vi "PixyCam_Open.vi"(4 "error in":errorcluster, 6 "SPI Bus":T4=enum."Invalid", 7 "Communication Mode":T5) -> (0 "error out":errorcluster, 3 "output cluster":T1)   [LabVIEW 2016, in "PixyCam_LabVIEW.lvlib"]
uses:
  PixyCam_LabVIEW.lvlib
  <vilib>/Rock Robotics/SystemInterfaces/spilib/spi_bus.ctl
  Private/PixyCam_CommMode.ctl
  Private/PixyCam_DevRef.ctl
  Private/PixyCam_SPI_DevRef.ctl
  <vilib>/Rock Robotics/WPI/SPI/WPI_SPIDevRef.ctl
  <vilib>/Rock Robotics/WPI/SPI/WPI_SPIMode.ctl
  <vilib>/Utility/SystemLogging/NI_SystemLogging.lvlib
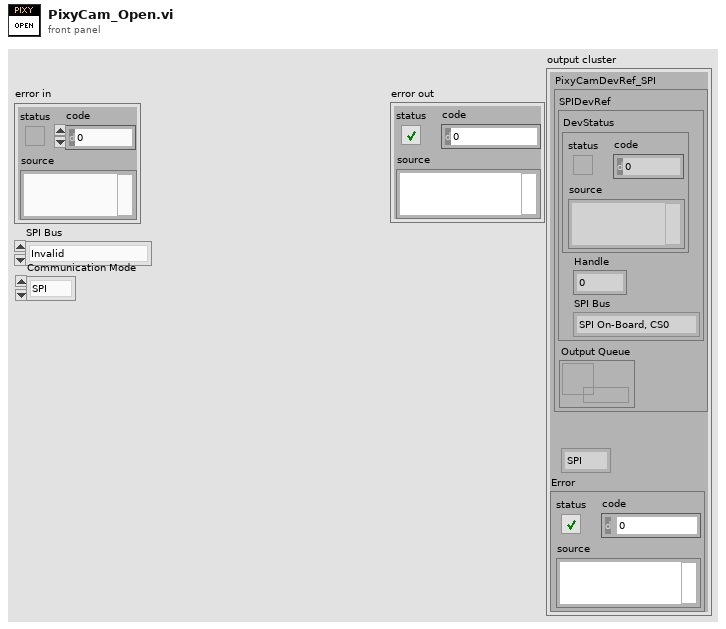
[diagram p1: front panel]
types:
  T1 = typedef "PixyCam_LabVIEW.lvlib/PixyCam_DevRef.ctl" = cluster{"PixyCamDevRef_SPI":T2, "Communication Mode":T5, "Error":errorcluster}
  T2 = typedef "PixyCam_LabVIEW.lvlib/PixyCam_SPI_DevRef.ctl" = cluster{"SPIDevRef":T3, "Output Queue":refnum<queue>}
  T3 = typedef "WPI_SPIDevRef.ctl" = cluster{"DevStatus":errorcluster, "Handle":i32, "SPI Bus":T4}
  T4 = typedef "spi_bus.ctl" = enum16{"SPI On-Board, CS0", "SPI On-Board, CS1", "SPI On-Board, CS2", "SPI On-Board, CS3", "SPI MXP", "Invalid"}
  T5 = typedef "PixyCam_LabVIEW.lvlib/PixyCam_CommMode.ctl" = enum16{"SPI", "I2C", "UART", "Analog", "Digital"}
  T6 = typedef "WPI_SPIMode.ctl" = enum16{"Mode 0 (Clk Idle Low,Sample on Leading)", "Mode 1 (Clk Idle Low,Sample on Trailing)", "Mode 2 (Clk Idle High,Sample on Leading)", "Mode 3 (Clk Idle High,Sample on Trailing)"}
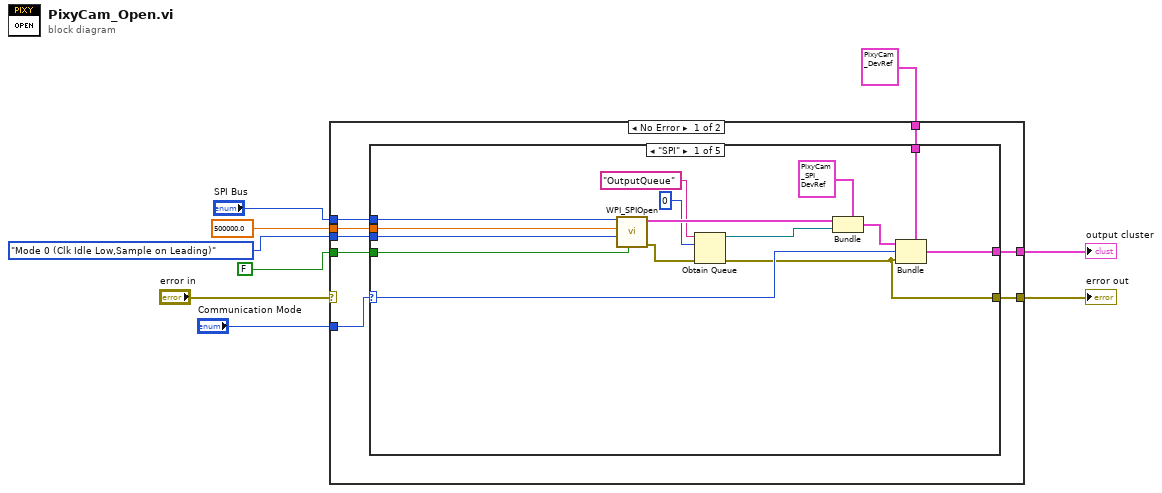
[diagram p0: block diagram]
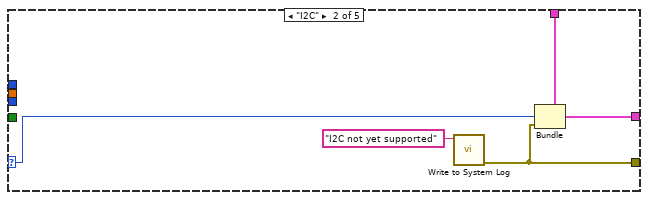
[diagram p2: hidden frame]
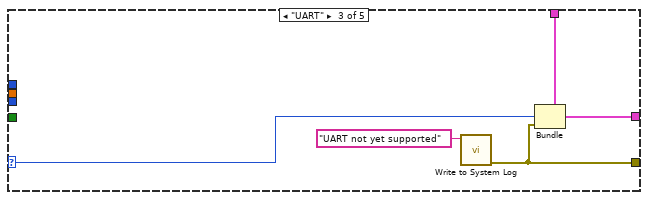
[diagram p3: hidden frame]
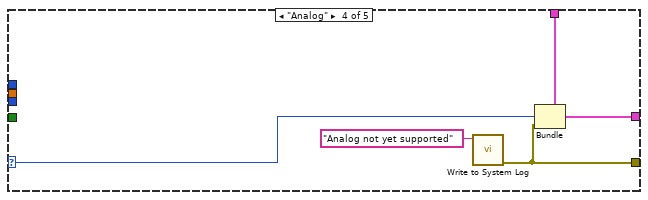
[diagram p4: hidden frame]
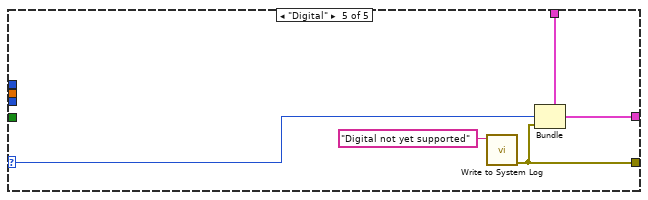
[diagram p5: hidden frame]
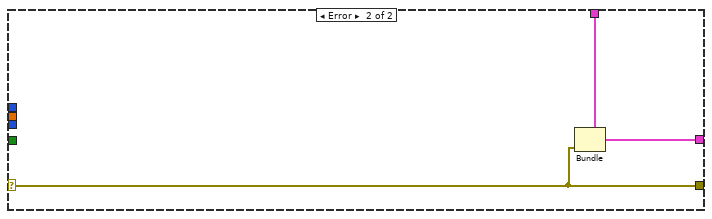
[diagram p6: hidden frame]
diagram:
  n1 = case shown="No Error" "error in" {
    selector: "error in" -> [_ w53]
    tunnel: [w12 w53] -> w8
    tunnel: 500000.0 ("Clock Rate (Hz)") -> [w17 _]
    tunnel: "SPI Bus" -> [w16 _]
    tunnel: WPI_SPIMode."Mode 0 (Clk Idle Low,Sample on Leading)" ("Mode (3)") -> [w15 _]
    tunnel: FALSE ("Chip Select Active High (F)") -> [w14 _]
    tunnel: "Communication Mode" -> [w13 _]
    tunnel: T1 {"PixyCamDevRef_SPI"={"SPIDevRef"={"DevStatus"={"status"=FALSE, "code"=0, "source"=""}, "Handle"=0, "SPI Bus"=enum."SPI On-Board, CS0"}, "Output Queue"=refnum}, "Communication Mode"=enum."SPI", "Error"={"status"=FALSE, "code"=0, "source"=""}} ("cluster") -> [w11 w54]
    tunnel: [w10 w55] -> w1
    frame No Error {
      n2 = case shown="\"SPI\"" w13 {
        selector: w13 -> [w27 w34 w38 w45 w48]
        tunnel: w17 -> [w32 _ _ _ _]
        tunnel: w16 -> [w31 _ _ _ _]
        tunnel: w15 -> [w30 _ _ _ _]
        tunnel: w14 -> [w29 _ _ _ _]
        tunnel: [w21 w33 w39 w44 w49] -> w12
        tunnel: w11 -> [w25 w36 w41 w46 w50]
        tunnel: [w24 w35 w40 w43 w51] -> w10
        frame "SPI" {
          n3 = call <vilib>:"WPI_SPIOpen.vi"("Chip Select Active High (F)"=w29, "Mode (3)"=w30, "Clock Rate (Hz)"=w32, "SPI Bus"=w31) -> ("error out"=w22:errorcluster, "SPIDevRef"=w28:T3)  [unwired: 6 in]
          n4 = Obtain Queue(name (unnamed)="OutputQueue", element data type=u8 0, error in (no error)=w22) -> (queue out=w18:refnum<queue>, error out=w21:errorcluster)  [unwired: 2 in, 1 out]
          n5 = Bundle(cluster=T2 {"SPIDevRef"={"DevStatus"={"status"=FALSE, "code"=0, "source"=""}, "Handle"=0, "SPI Bus"=enum."SPI On-Board, CS0"}, "Output Queue"=refnum}, "SPIDevRef"=w28, "Output Queue"=w18) -> (w26:T2)
          n6 = Bundle(cluster=w25, "PixyCamDevRef_SPI"=w26, "Communication Mode"=w27, "Error"=w21) -> (w24:T1)
        }
        frame "I2C" {
          n7 = call <vilib>:"Write to System Log.vi"("message"="I2C not yet supported") -> ("error out"=w33:errorcluster)  [unwired: 10 in]
          n8 = Bundle(cluster=w36, "Communication Mode"=w34, "Error"=w33) -> (w35:T1)  [unwired: 1 in]
        }
        frame "UART" {
          n9 = call <vilib>:"Write to System Log.vi"("message"="UART not yet supported") -> ("error out"=w39:errorcluster)  [unwired: 10 in]
          n10 = Bundle(cluster=w41, "Communication Mode"=w38, "Error"=w39) -> (w40:T1)  [unwired: 1 in]
        }
        frame "Analog" {
          n11 = call <vilib>:"Write to System Log.vi"("message"="Analog not yet supported") -> ("error out"=w44:errorcluster)  [unwired: 10 in]
          n12 = Bundle(cluster=w46, "Communication Mode"=w45, "Error"=w44) -> (w43:T1)  [unwired: 1 in]
        }
        frame "Digital" {
          n13 = call <vilib>:"Write to System Log.vi"("message"="Digital not yet supported") -> ("error out"=w49:errorcluster)  [unwired: 10 in]
          n14 = Bundle(cluster=w50, "Communication Mode"=w48, "Error"=w49) -> (w51:T1)  [unwired: 1 in]
        }
      }
    }
    frame Error {
      n15 = Bundle(cluster=w54, "Error"=w53) -> (w55:T1)  [unwired: 2 in]
    }
  }
  "error out" <- w8
  "output cluster" <- w1
